vi "Read Frequencies and Amplitudes.vi"(8 "error in (no error)":errorcluster, 11 "SV Discrete Sweep in":refnum<class "SV Discrete Sweep.lvclass">) -> (0 "error out":errorcluster, 1 "amplitudes":dbl[](array[numeric]), 2 "frequencies_Hz":dbl[](array[numeric]), 3 "SV Discrete Sweep out":refnum<class "SV Discrete Sweep.lvclass">, 4 "number of steps":i32)   [LabVIEW 2017, in "SV Discrete Sweep.lvclass"]
uses:
  <vilib>/addons/_NISVFA/_Generation/Signal Generation/SV Discrete Sweep/SV Discrete Sweep.lvclass
  <vilib>/addons/_NISVFA/_Generation/Signal Generation/SV Discrete Sweep/SV Discrete Sweep.lvclass/SV Discrete Sweep.ctl
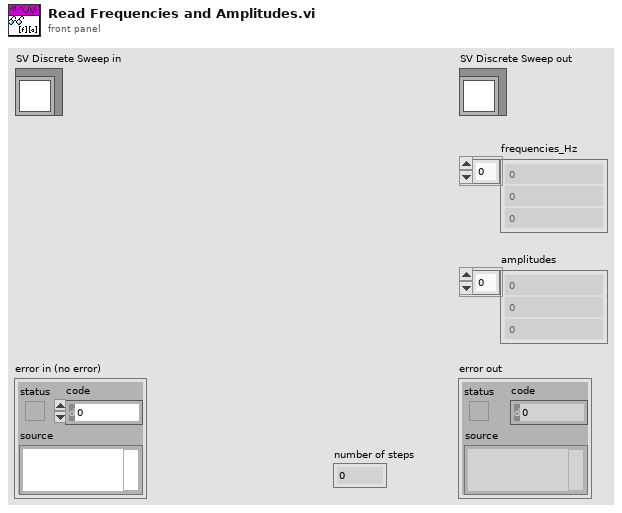
[diagram p1: front panel]
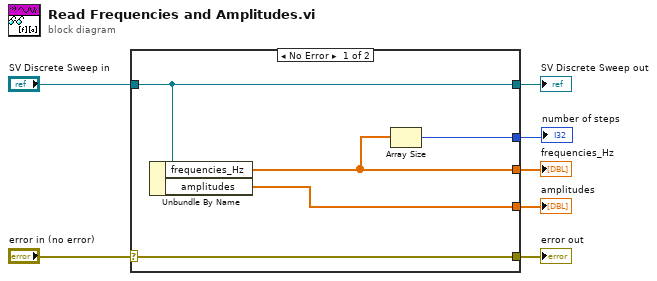
[diagram p0: block diagram]
diagram:
  n1 = case shown="No Error" "error in (no error)" {
    selector: "error in (no error)" -> [w12 w13]
    tunnel: [w12 w13] -> w6
    tunnel: [w11 w14] -> w4
    tunnel: "SV Discrete Sweep in" -> [w11 w14]
    tunnel: [w9 _] -> w3
    tunnel: [w10 _] -> w2
    tunnel: [w8 _] -> w1
    frame No Error {
      n2 = Unbundle By Name(w11) -> ("frequencies_Hz"=w9:dbl[], "amplitudes"=w10:dbl[])
      n3 = Array Size(array=w9) -> (size(s)=w8:i32)
    }
    frame Error {
    }
  }
  "error out" <- w6
  "SV Discrete Sweep out" <- w4
  "frequencies_Hz" <- w3
  "amplitudes" <- w2
  "number of steps" <- w1
